vi "Basic Input Demo.vi"() -> ()   [LabVIEW 2013]
doc: "This VI show how to use the basic functions in the Input Device palette. It will show information about all the joysticks, keyboards and mice attached to the system (number of axes, buttons, pov, and the name). It will also give the current information for the first joystick attached to the system (location and button pressed). The current information for the first keyboard and mouse will also be displayed."
uses:
  <vilib>/Utility/inputDevices.llb/closeMouse.vi
  <vilib>/Utility/inputDevices.llb/closeKeyboard.vi
  <vilib>/Utility/inputDevices.llb/mouseAcquire.vi
  <vilib>/Utility/inputDevices.llb/keyboardAcquire.vi
panel:
  in  "keyboard loop (ms)":u32=200
  in  "mouse loop (ms)":u32=100
  in  "keyboard service name":string="/keyboard"
  in  "mouse service name":string="/mouse"
  out "caps on":bool
  out "ADDRESS":string
  in  "mode":T1(ring)=enum."Write"
  out "DATASOCKET DETAILS FOR MOUSE":string="dstp://xxxxx/mouse"
  out "MOUSE INFO":T2
  out "x .or. y?":bool
  out "mouse data":string
  out "Mouse Bytes":i32
  out "Middle Button Pressed":bool
  out "Right Button Pressed":bool
  out "Left Button Pressed":bool
  out "Axis Info":T3
  out "Mouse Info":T4(array[cluster])
  out "Keys Pressed":T5(array[ring])
  out "Key Info":T6(array[cluster])
  in  "stop":bool
  # "COPY THIS ADDRESS TO CLIENT MACHINE"
  # "KEYBOARD/KEYPADS"
  # "MICE"
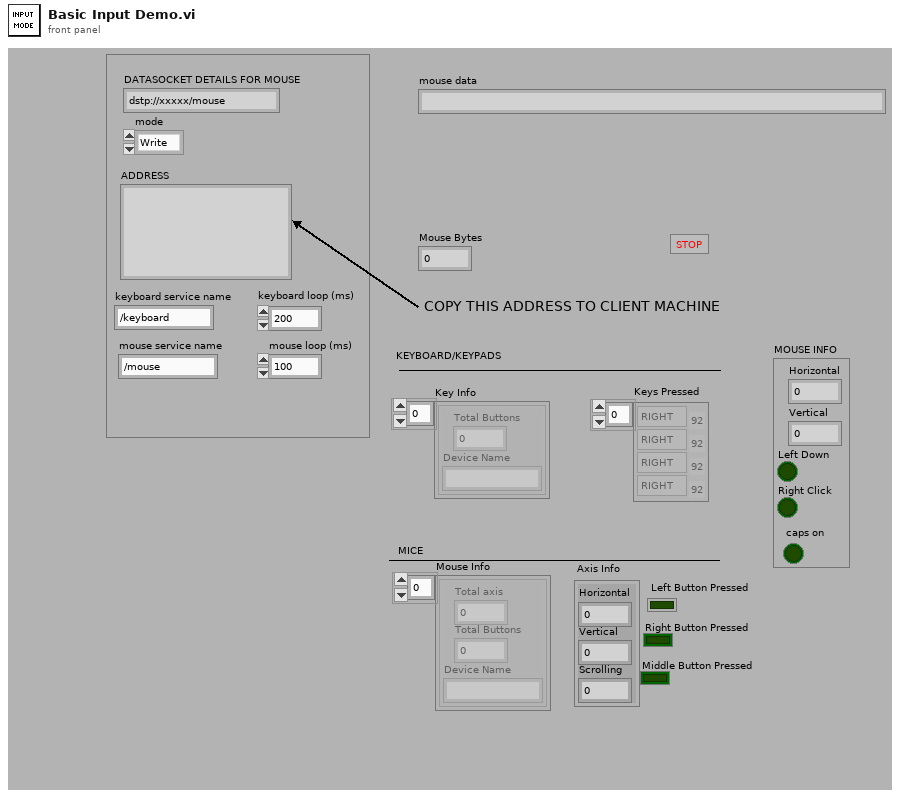
[diagram p1: front panel]
types:
  T1 = enum16{"Read", "Write", "ReadWrite", "BufferedRead", "BufferedReadWrite"}
  T2 = cluster{"Horizontal":i32, "Vertical":i32, "Left Down":bool, "Right Click":bool, "caps on":bool}
  T3 = cluster{"Horizontal":i32, "Vertical":i32, "Scrolling":i32}
  T4 = cluster{"Total axis":u32, "Total Buttons":u32, "Device Name":string}[]
  T5 = enum16{"0", "1", "2", "3", "4", "5", "6", "7", "8", "9", "A", "B", "C", "D", "E", "F", "G", "H", "I", "J", "K", "L", "M", "N", "O", "P", "Q", "R", "S", "T", "U", "V", "W", "X", "Y", "Z", "F1", "F2", "F3", "F4", "F5", "F6", "F7", "F8", "F9", "F10", "F11", "F12", "F13", "F14", "F15", "ADD", "BACK", "BACKSLASH", "CAPITAL", "COMMA", "DECIMAL", "DELETE", "DIVIDE", "DOWN", "END", "EQUALS", "ESCAPE", "GRAVE (`)", "HOME", "INSERT", "LBRACKET", "LCONTROL", "LEFT", "L ALT", "LSHIFT", "LWIN", "MINUS", "MULTIPLY", "NEXT", "NUMLOCK", "NUMPAD_0", "NUMPAD_1", "NUMPAD_2", "NUMPAD_3", "NUMPAD_4", "NUMPAD_5", "NUMPAD_6", "NUMPAD_7", "NUMPAD_8", "NUMPAD_9", "PAUSE", "PERIOD", "PRIOR (PG UP)", "RBRACKET", "RCONTROL", "RETURN", "RIGHT", "R ALT", "RSHIFT", "RWIN", "SCROLL", "SEMICOLON", "SLASH", "SPACE", "SUBTRACT", "TAB", "UP", "ENTER (num pad)", "' (quote)"}[]
  T6 = cluster{"Total Buttons":u32, "Device Name":string}[]
  T7 = cluster{"Axis Info 2":cluster{"Horizontal":i32, "Vertical":i32, "Scrolling":i32}, "button info":cluster{"button 1":bool, "button 2":bool, "button 3":bool, "button 4":bool}}
  T8 = cluster{"axes total":u32, "buttons total":u32, "device name":string}[]
  T9 = cluster{"buttons total":u32, "device name":string}[]
  T10 = enum16{"0", "1", "2", "3", "4", "5", "6", "7", "8", "9", "A", "B", "C", "D", "E", "F", "G", "H", "I", "J", "K", "L", "M", "N", "O", "P", "Q", "R", "S", "T", "U", "V", "W", "X", "Y", "Z", "F1", "F2", "F3", "F4", "F5", "F6", "F7", "F8", "F9", "F10", "F11", "F12", "F13", "F14", "F15", "ADD", "BACK", "BACKSLASH", "CAPITAL", "COMMA", "DECIMAL", "DELETE", "DIVIDE", "DOWN", "END", "EQUALS", "ESCAPE", "GRAVE (`)", "HOME", "INSERT", "LBRACKET", "LCONTROL", "LEFT", "L ALT", "LSHIFT", "LWIN", "MINUS", "MULTIPLY", "NEXT", "NUMLOCK", "NUMPAD_0", "NUMPAD_1", "NUMPAD_2", "NUMPAD_3", "NUMPAD_4", "NUMPAD_5", "NUMPAD_6", "NUMPAD_7", "NUMPAD_8", "NUMPAD_9", "PAUSE", "PERIOD", "PRIOR (PG UP)", "RBRACKET", "RCONTROL", "RETURN", "RIGHT", "R ALT", "RSHIFT", "RWIN", "SCROLL", "SEMICOLON", "SLASH", "SPACE", "SUBTRACT", "TAB", "UP", "ENTER (num pad)", "' (quote)"}
  T11 = cluster{"button 1":bool, "button 2":bool, "button 3":bool, "button 4":bool}
  T12 = cluster{"Horizontal":i32, "Vertical":i32, "button 1":bool, "button 2":bool, "caps on":bool}
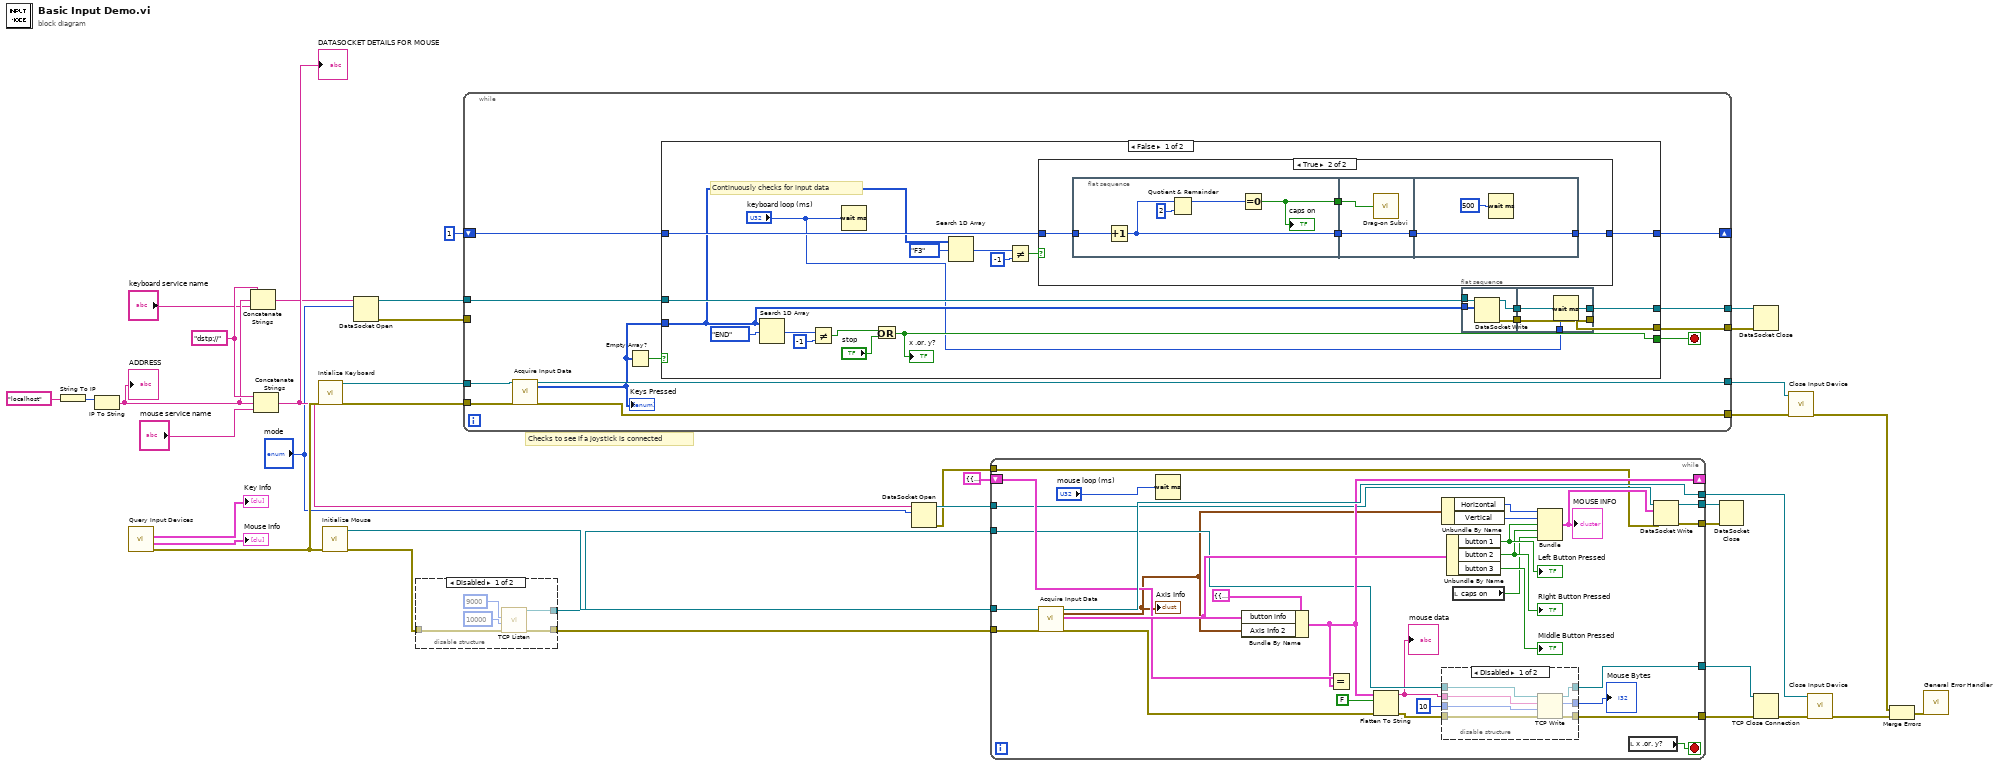
[diagram p0: block diagram]
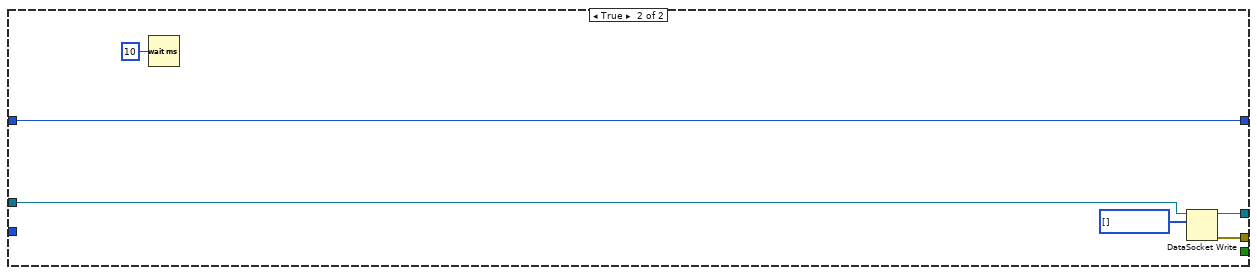
[diagram p5: hidden frame]
diagram:
  w11 = "dstp://" ("string")
  # "Checks to see if a joystick is connected"
  n1 = String To IP(1:"localhost" ("name")) -> (0:w14:u32)
  n2 = IP To String(2:w14) -> (0:w10:string)  [unwired: 1 in]
  "ADDRESS" <- w10
  n3 = call <vilib>:"Query Input Devices.vi"() -> ("error out"=w35:errorcluster, "mouse info"=→"Mouse Info":T8, "key info"=→"Key Info":T9)  [unwired: 8 in, 1 out]
  n4 = Concatenate Strings(w11, w10, "keyboard service name") -> (w8:string)
  n5 = Concatenate Strings(w11, w10, "mouse service name") -> (w12:string)
  "DATASOCKET DETAILS FOR MOUSE" <- w12
  n6 = call <vilib>:"Intialize Keyboard.vi"("error in (no error)"=w35) -> ("error out"=w36:errorcluster, "device ID"=w37:refnum<k1>)  [unwired: 9 in]
  n7 = call <vilib>:"Initialize Mouse.vi"("error in (no error)"=w35) -> ("error out"=w21:errorcluster, "device ID"=w28:refnum<k1>)  [unwired: 9 in]
  n8 = DataSocket Open(10:"mode", 11:w8) -> (0:w5:errorcluster, 3:w6:refnum<k13>)  [unwired: 2 in]
  n9 = disable-structure shown="Disabled" {
    disable-tunnel: [w40 _] -> w27
    disable-tunnel: [w39 _] -> w26
    disable-tunnel: w21 -> [w38 _]
    frame Disabled {
      n10 = call <vilib>:"TCP Listen.vi"("error in (no error)"=w38, "timeout ms (wait forever: -1)"=10000, "port"=u16 9000) -> ("error out"=w40:errorcluster, "connection ID"=w39:refnum<k5>)  [unwired: 4 in, 3 out]
    }
    frame Enabled {
    }
  }
  n11 = while {
    tunnel: w37 -> [w54]
    tunnel: w36 -> [w53]
    tunnel: [w52] -> w31
    tunnel: [w51] -> w20
    tunnel: w6 -> [w48]
    tunnel: w5 -> [_]
    shift-right: [w50] -> _
    shift-left: 1 -> [w49]
    tunnel: [w47] -> w3
    tunnel: [w46] -> w2
    stop <- w43 stop-if-true
    n12 = call-poly <vilib>:"Acquire Input Data.vi"("device ID"=w54, "error in (no error)"=w53) -> ("device ID"=w52:refnum<k1>, "keys pressed"=w45:T5, "error out"=w51:errorcluster)  [unwired: 15 in]
    "Keys Pressed" <- w45
    n13 = Empty Array?(array=w45) -> (empty?=w44:bool)
    n14 = case shown="False" w44 {
      tunnel: [w73 _] -> w43
      tunnel: [w64 w101] -> w50
      tunnel: w49 -> [w63 w101]
      tunnel: w48 -> [w62 w98]
      tunnel: [w60 w100] -> w47
      tunnel: [w59 w99] -> w46
      tunnel: w45 -> [w58 _]
      frame False {
        # "Continuously checks for input data"
        n15 = Search 1D Array(1D array=w58, element=T10."END" ("keyType 3")) -> (index of element=w71:i32)  [unwired: 1 in]
        n16 = Not Equal?(x=w71, y=-1) -> (x != y?=w69:bool)
        n17 = Wait (ms)(milliseconds to wait="keyboard loop (ms)") -> ()  [unwired: 1 out]
        n18 = Or(x=w69, y="stop") -> (x .or. y?=w73:bool)
        "x .or. y?" <- w73
        n19 = Search 1D Array(1D array=w58, element=T10."F3" ("keyType 3")) -> (index of element=w66:i32)  [unwired: 1 in]
        n20 = Not Equal?(x=w66, y=-1) -> (x != y?=w65:bool)
        n21 = case shown="True" w65 {
          tunnel: w63 -> [w81 w86]
          tunnel: [w81 w85] -> w64
          frame False {
          }
          frame True {
            n22 = flat-sequence {
              tunnel: w86 -> [w91]
              tunnel: [w90] -> w84
              tunnel: [w87] -> w82
              tunnel: w84 -> [w93]
              tunnel: [w93] -> w83
              tunnel: w82 -> [w92]
              tunnel: [w95] -> w85
              tunnel: w83 -> [w95]
              frame #0 {
                n23 = Increment(x=w91) -> (x+1=w90:i32)
                n24 = Quotient & Remainder(x=w90, y=2) -> (x-y*floor(x/y)=w88:i32)  [unwired: 1 out]
                n25 = Equal To 0?(x=w88) -> (x = 0?=w87:bool)
                "caps on" <- w87
              }
              frame #1 {
                n26 = call "Drag-on Subvi.vi"(w92) -> ()
              }
              frame #2 {
                n27 = Wait (ms)(milliseconds to wait=u32 500) -> ()  [unwired: 1 out]
              }
            }
          }
        }
        n28 = flat-sequence {
          tunnel: w62 -> [w77]
          tunnel: w58 -> [w74]
          tunnel: [w76] -> w57
          tunnel: [w75] -> w56
          tunnel: [w79] -> w59
          tunnel: [w80] -> w60
          tunnel: w57 -> [w80]
          tunnel: w56 -> [w79]
          tunnel: "keyboard loop (ms)" -> [w78]
          frame #0 {
            n29 = DataSocket Write(10:w74, 11:w77) -> (0:w75:errorcluster, 3:w76:refnum<k13>)  [unwired: 2 in, 1 out]
          }
          frame #1 {
            n30 = Wait (ms)(milliseconds to wait=w78) -> ()  [unwired: 1 out]
          }
        }
      }
      frame True {
        w97 = T5 [] items=["0", "1", "2", "3", "4", "5", "6", "7", "8", "9", "A", "B", "C", "D", "E", "F", "G", "H", "I", "J", "K", "L", "M", "N", "O", "P", "Q", "R", "S", "T", "U", "V", "W", "X", "Y", "Z", "F1", "F2", "F3", "F4", "F5", "F6", "F7", "F8", "F9", "F10", "F11", "F12", "F13", "F14", "F15", "ADD", "BACK", "BACKSLASH", "CAPITAL", "COMMA", "DECIMAL", "DELETE", "DIVIDE", "DOWN", "END", "EQUALS", "ESCAPE", "GRAVE (`)", "HOME", "INSERT", "LBRACKET", "LCONTROL", "LEFT", "L ALT", "LSHIFT", "LWIN", "MINUS", "MULTIPLY", "NEXT", "NUMLOCK", "NUMPAD_0", "NUMPAD_1", "NUMPAD_2", "NUMPAD_3", "NUMPAD_4", "NUMPAD_5", "NUMPAD_6", "NUMPAD_7", "NUMPAD_8", "NUMPAD_9", "PAUSE", "PERIOD", "PRIOR (PG UP)", "RBRACKET", "RCONTROL", "RETURN", "RIGHT", "R ALT", "RSHIFT", "RWIN", "SCROLL", "SEMICOLON", "SLASH", "SPACE", "SUBTRACT", "TAB", "UP", "ENTER (num pad)", "' (quote)"] ("keys pressed")
        n31 = Wait (ms)(milliseconds to wait=u32 10) -> ()  [unwired: 1 out]
        n32 = DataSocket Write(10:w97, 11:w98) -> (0:w99:errorcluster, 3:w100:refnum<k13>)  [unwired: 2 in, 1 out]
      }
    }
  }
  n33 = DataSocket Open(10:"mode", 11:w12) -> (0:w1:errorcluster, 3:w18:refnum<k13>)  [unwired: 2 in]
  n34 = while {
    tunnel: w28 -> [w130]
    tunnel: w27 -> [w129]
    tunnel: w26 -> [w118]
    tunnel: [w119] -> w25
    tunnel: [w120] -> w24
    tunnel: [w124] -> w23
    shift-right: [w121] -> _
    shift-left: T7 {"Axis Info 2"={"Horizontal"=0, "Vertical"=0, "Scrolling"=0}, "button info"={"button 1"=FALSE, "button 2"=FALSE, "button 3"=FALSE, "button 4"=FALSE}} ("button info") -> [w123]
    tunnel: w18 -> [w117]
    tunnel: [w116] -> w17
    tunnel: [w115] -> w16
    tunnel: w1 -> [w102]
    stop <- w126 stop-if-true
    n35 = call-poly <vilib>:"Acquire Input Data.vi"("device ID"=w130, "error in (no error)"=w129) -> ("device ID"=w124:refnum<k1>, "axis info"=w114:T3, "button info"=w127:T11, "error out"=w122:errorcluster)  [unwired: 14 in]
    "Axis Info" <- w114
    n36 = Wait (ms)(milliseconds to wait="mouse loop (ms)") -> ()  [unwired: 1 out]
    n37 = Bundle By Name(cluster=T7 {"Axis Info 2"={"Horizontal"=894, "Vertical"=768, "Scrolling"=0}, "button info"={"button 1"=FALSE, "button 2"=FALSE, "button 3"=FALSE, "button 4"=FALSE}} ("button info"), "button info"=w127, "Axis Info 2"=w114) -> (w121:T7)
    n38 = Equal?(x=w123, y=w121) -> ()  [unwired: 1 out]
    n39 = Flatten To String(anything=w121, prepend array or string size? (T)=FALSE, error in (no error)=w122) -> (data string=w105:string, error out=w106:errorcluster)  [unwired: 1 in, 1 out]
    "mouse data" <- w105
    n40 = Unbundle By Name(w114) -> ("Horizontal"=w113:i32, "Vertical"=w112:i32)
    n41 = disable-structure shown="Disabled" {
      disable-tunnel: w105 -> [w138 _]
      disable-tunnel: 10 ("timeout ms (25000)") -> [w137 _]
      disable-tunnel: [w136 _] -> w107
      disable-tunnel: w106 -> [w135 _]
      disable-tunnel: [w134 _] -> w120
      disable-tunnel: [w133 _] -> w119
      disable-tunnel: w118 -> [w132 _]
      frame Disabled {
        n42 = TCP Write(connection ID=w132, data in=w138, error in (no error)=w135, 9:w137) -> (connection ID out=w133:refnum<k5>, bytes written=w136:i32, error out=w134:errorcluster)
      }
      frame Enabled {
      }
    }
    "Mouse Bytes" <- w107
    n43 = Unbundle By Name(w127) -> ("button 1"=w111:bool, "button 2"=w110:bool, "button 3"=→"Middle Button Pressed":bool)
    "Left Button Pressed" <- w111
    "Right Button Pressed" <- w110
    n44 = local read "caps on"() -> (w104:bool)
    n45 = Bundle("Horizontal"=w113, "Vertical"=w112, "button 1"=w111, "button 2"=w110, "caps on"=w104) -> (w103:T12)  [unwired: 1 in]
    "MOUSE INFO" <- w103
    n46 = local read "x .or. y?"() -> (w126:bool)
    n47 = DataSocket Write(8:w102, 10:w103, 11:w117) -> (0:w115:errorcluster, 3:w116:refnum<k13>)  [unwired: 1 in, 1 out]
  }
  n48 = DataSocket Close(8:w16, 11:w17) -> ()  [unwired: 1 in, 2 out]
  n49 = DataSocket Close(8:w2, 11:w3) -> ()  [unwired: 1 in, 2 out]
  n50 = TCP Close Connection(connection ID=w25, error in (no error)=w24) -> (error out=w22:errorcluster)  [unwired: 1 in, 1 out]
  n51 = call-poly <vilib>:"Close Input Device.vi"("error in (no error)"=w20, "device ID"=w31) -> ("error out"=w29:errorcluster)  [unwired: 8 in]
  n52 = call-poly <vilib>:"Close Input Device.vi"("error in (no error)"=w22, "device ID"=w23) -> ("error out"=w30:errorcluster)  [unwired: 8 in]
  n53 = Merge Errors(w29, w30) -> (w32:errorcluster)
  n54 = call <vilib>:"General Error Handler.vi"("error in (no error)"=w32) -> ()  [unwired: 10 in, 5 out]
